vi "WinCI Remove.vi"(7 "advanced options":variant, 8 "error in (no error)":errorcluster, 9 "comment":string, 10 "files":path[](array[path]), 11 "source control reference in":T1) -> (0 "error out":errorcluster, 1 "dialog box cancelled?":bool, 2 "status message":string, 3 "source control reference out":T1)   [LabVIEW 2020, in "NI_SCC_WinCI.lvlib"]
uses:
  <vilib>/SourceControl/Providers/WinCI/NI_SCC_WinCI.lvlib
  <vilib>/SourceControl/sccapi/SCCAPI Refnum.ctl
  <vilib>/SourceControl/support/SCCSup Message Strings GLBL.vi
  <vilib>/SourceControl/sccapi/NI_SCC.lvlib
panel:
  out "result":i32
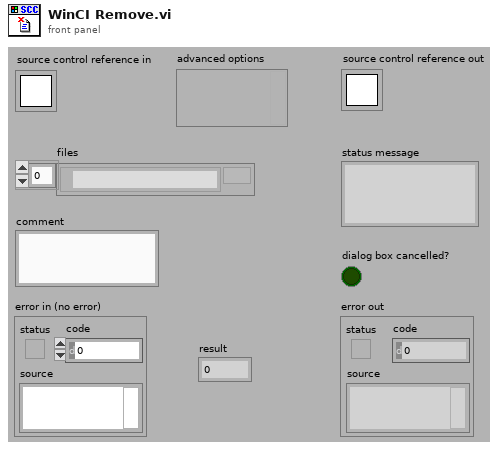
[diagram p1: front panel]
types:
  T1 = typedef "NI_SCC.lvlib/SCCAPI Refnum.ctl" = refnum<k1>
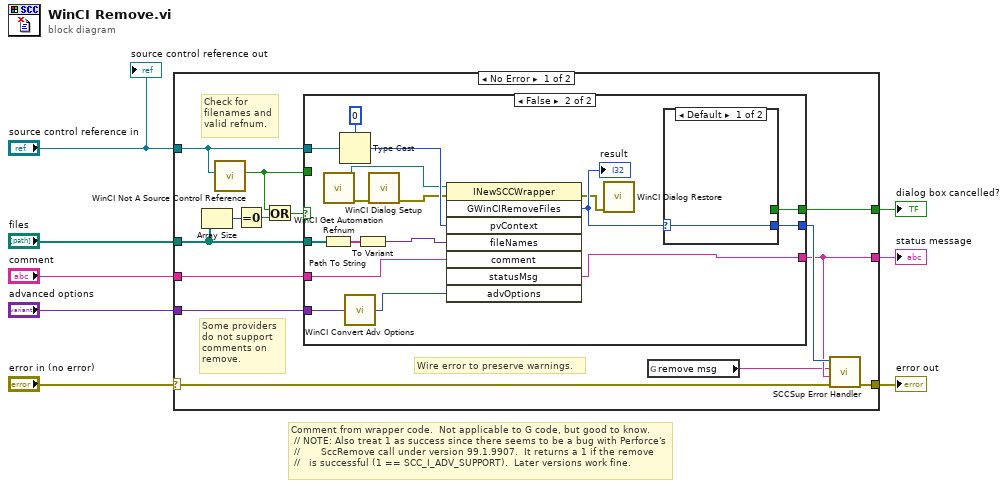
[diagram p0: block diagram]
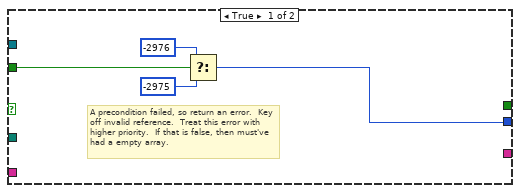
[diagram p2: hidden frame]
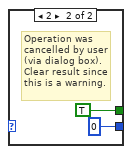
[diagram p3: hidden frame]
diagram:
  # "Comment from wrapper code.  Not applicable to G code, but good to know.\n\t// NOTE: Also treat 1 as success since there seems to be a bug with Perforce's\n\t//       SccRemove call under version 99.1.9907.  It returns a 1 if the remove\n\t//\t\t is successful (1 == SCC_I_ADV_SUPPORT).  Later versions work fine."
  n1 = case shown="No Error" "error in (no error)" {
    selector: "error in (no error)" -> [w17 w47]
    tunnel: [w21 w47] -> w7
    tunnel: "source control reference in" -> [w9 _]
    tunnel: [w19 _] -> w5
    tunnel: "files" -> [w14 _]
    tunnel: "comment" -> [w22 _]
    tunnel: [w12 _] -> w2
    tunnel: "advanced options" -> [w11 _]
    frame No Error {
      # "Check for filenames and valid refnum."
      # "Some providers do not support comments on remove."
      # "Wire error to preserve warnings."
      n2 = Array Size(array=w14) -> (size(s)=w16:i32)
      n3 = call <vilib>:"WinCI Not A Source Control Reference.vi"("source control reference in"=w9) -> ("not a source control reference?"=w10:bool)  [unwired: 1 in, 9 out]
      n4 = Equal To 0?(x=w16) -> (x = 0?=w15:bool)
      n5 = Or(x=w10, y=w15) -> (x .or. y?=w13:bool)
      n6 = case shown="False" w13 {
        tunnel: w9 -> [_ w43]
        tunnel: [_ w36] -> w19
        tunnel: w14 -> [_ w41]
        tunnel: w22 -> [_ w34]
        tunnel: [w23 w40] -> w20
        tunnel: w10 -> [w24 _]
        tunnel: [_ w39] -> w12
        tunnel: w11 -> [_ w38]
        frame True {
          # "A precondition failed, so return an error.  Key off invalid reference.  Treat this error with higher priority.  If that is false, then must've had a empty array."
          n7 = Select(t=-2976 ("result"), s=w24, f=-2975 ("result")) -> (s? t:f=w23:i32)
        }
        frame False {
          n8 = Path To String(path=w41) -> (string=w31:string[])
          n9 = call <vilib>:"WinCI Get Automation Refnum.vi"() -> ("error out"=w29:errorcluster, "automation refnum"=w30:refnum<k7>)  [unwired: 10 out]
          n10 = Type Cast(type=u32 0, x=w43) -> (*(type *) &x=w33:u32)
          n11 = call <vilib>:"WinCI Convert Adv Options.vi"("advanced options"=w38) -> ("command options"=w35:u32)  [unwired: 4 out]
          n12 = To Variant(anything=w31) -> (Variant=w32:variant)
          n13 = call <vilib>:"WinCI Dialog Setup.vi"("error in"=w29) -> ("error out"=w28:errorcluster)  [unwired: 10 out]
          n14 = invoke class="INewSCCWrapper" method="GWinCIRemoveFiles"(reference=w30, error in=w28, "pvContext"=w33, "fileNames"=w32, "comment"=w34, "advOptions"=w35) -> (error out=w27:errorcluster, "GWinCIRemoveFiles"=w37:i32, "statusMsg"=w36:string)  [unwired: 2 in, 5 out]
          "result" <- w37
          n15 = call <vilib>:"WinCI Dialog Restore.vi"("error in"=w27) -> ()  [unwired: 11 out]
          n16 = case shown="Default" w37 {
            selector: w37 -> [w44 _]
            tunnel: [w44 0 ("result")] -> w40
            tunnel: [_ TRUE] -> w39
            frame Default {
            }
            frame 2 {
              # "Operation was cancelled by user (via dialog box).  Clear result since this is a warning."
            }
          }
        }
      }
      n17 = global read "SCCSup Message Strings GLBL.vi" "remove msg"() -> (w18:string)
      n18 = call <vilib>:"SCCSup Error Handler.vi"("error in (no error)"=w17, "additional message"=w19, "operation message"=w18, "scc error code"=w20) -> ("error out"=w21:errorcluster)  [unwired: 7 out]
    }
    frame Error {
    }
  }
  "error out" <- w7
  "status message" <- w5
  "dialog box cancelled?" <- w2
  "source control reference out" <- "source control reference in"
